vi "Write String.vi"(10 "string":string) -> (3 "String With Equals":refnum<class "String With Equals.lvclass">)   [LabVIEW 2023, in "String With Equals.lvclass"]
uses:
  String With Equals.lvclass
  String With Equals.lvclass/String With Equals.ctl
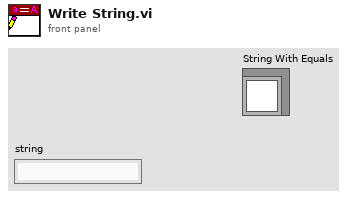
[diagram p1: front panel]
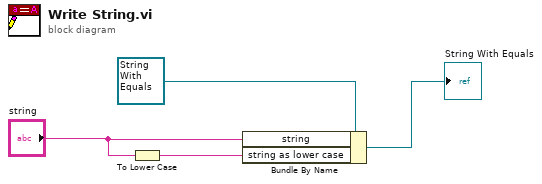
[diagram p0: block diagram]
diagram:
  n1 = To Lower Case(string="string") -> (all lower case string=w1:string)
  n2 = Bundle By Name(cluster=refnum<class "String With Equals.lvclass"> refnum ("String With Equals in"), "string"="string", "string as lower case"=w1) -> (→"String With Equals":refnum<class "String With Equals.lvclass">)
